vi "Graph AddCursor(Mixed).vi"(8 "エラー入力（エラーなし）":errorcluster, 9 "色":u32(colorbox), 10 "名称":string, 11 "MixedGraph入力":refnum<vi>) -> (0 "エラー出力":errorcluster)   [LabVIEW 2014]
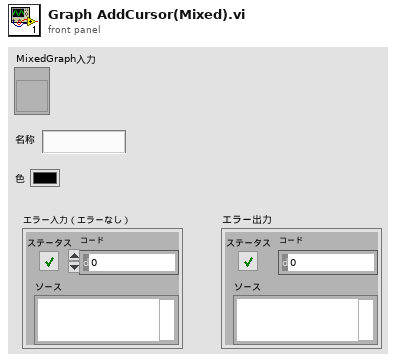
[diagram p1: front panel]
types:
  T1 = cluster{"Name":string, "Color":u32, "Style":u8, "Point Style":u8, "Name Visible":bool, "Allow Drag":bool, "Cursor Mode":u32, "Plot":i32, "Index":i32, "Position":cluster{"X":dbl, "Y":dbl}, "X Scale":u32, "Y Scale":u32, "Watch Plots":i32[], "Watch All Plots":bool, "Plot Area":i32, "Label Offset":cluster{"X":dbl, "Y":dbl}}
  T2 = typedef "LVCursorListTypeDef.ctl" = cluster{"Name":string, "Color":u32, "Style":u8, "Point Style":u8, "Name Visible":bool, "Allow Drag":bool, "Cursor Mode":u32, "Plot":i32, "Index":i32, "Position":cluster{"X":dbl, "Y":dbl}, "X Scale":u32, "Y Scale":u32, "Watch Plots":i32[], "Watch All Plots":bool, "Plot Area":i32, "Label Offset":cluster{"X":dbl, "Y":dbl}}[]
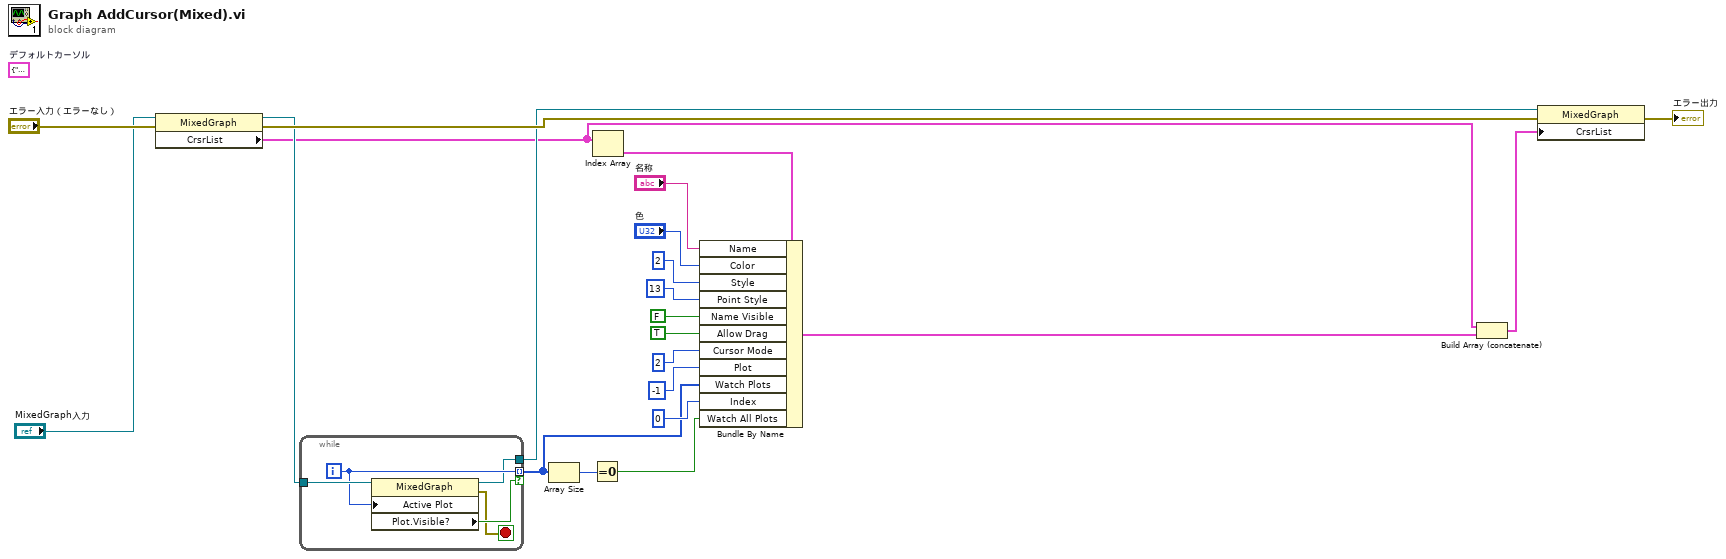
[diagram p0: block diagram]
diagram:
  (unwired) T1 {"Name"="カーソル0", "Color"=16776960, "Style"=2, "Point Style"=13, "Name Visible"=FALSE, "Allow Drag"=TRUE, "Cursor Mode"=2, "Plot"=-1, "Index"=42, "Position"={"X"=0.42, "Y"=43.0}, "X Scale"=0, "Y Scale"=0, "Watch Plots"=[], "Watch All Plots"=TRUE, "Plot Area"=0, "Label Offset"={"X"=-0.0012080536912751905, "Y"=172.10516252390056}}  # デフォルトカーソル
  n1 = property class="MixedGraph"(reference="MixedGraph入力", error in="エラー入力（エラーなし）") -> (reference out=w12:refnum<vi>, error out=w17:errorcluster, "CrsrList"=w2:T2)
  n2 = while {
    tunnel: w12 -> [w27]
    tunnel: [w26] -> w10 mode=indexing if=w25
    tunnel: [w24] -> w13
    i -> [w26]
    stop <- w23 stop-if-true
    n3 = property class="MixedGraph"(reference=w27, "Active Plot"=w26) -> (reference out=w24:refnum<vi>, error out=w23:errorcluster, "Plot.Visible?"=w25:bool)  [unwired: 1 in]
  }
  n4 = Array Size(array=w10) -> (size(s)=w9:i32)
  n5 = Equal To 0?(x=w9) -> (x = 0?=w8:bool)
  n6 = Index Array(array=w2) -> (element=w1:T1)  [unwired: 1 in]
  n7 = Bundle By Name(cluster=w1, "Name"="名称", "Color"="色", "Style"=u8 2, "Point Style"=u8 13, "Name Visible"=FALSE, "Allow Drag"=TRUE, "Cursor Mode"=u32 2, "Plot"=-1, "Watch Plots"=w10, "Index"=0, "Watch All Plots"=w8) -> (w14:T1)
  n8 = Build Array (concatenate)(w2, w14) -> (w19:T2)
  n9 = property class="MixedGraph"(reference=w13, error in=w17, "CrsrList"=w19) -> (error out=→"エラー出力":errorcluster)  [unwired: 1 out]
